vi "DAQinfo.vi"() -> (0 "错误？":bool, 1 "错误信息":string, 2 "DaqSn":string, 3 "DeviceNO":tag)   [LabVIEW 2010]
uses:
  C:/Program Files (x86)/National Instruments/LabVIEW 2010/resource/objmgr/daqmx.rc
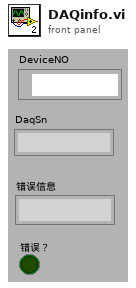
[diagram p1: front panel]
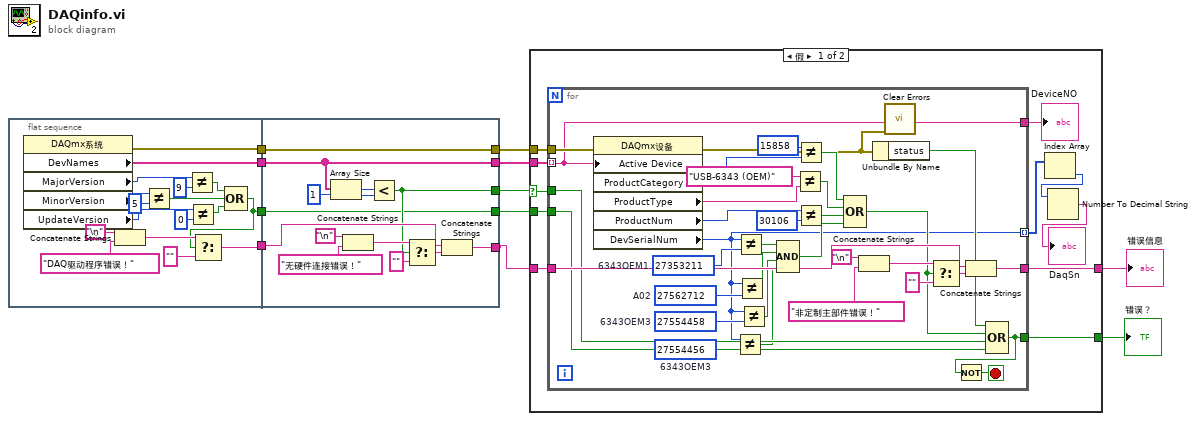
[diagram p0: block diagram]
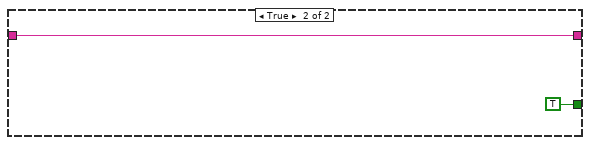
[diagram p2: hidden frame]
diagram:
  n1 = flat-sequence {
    tunnel: [w28] -> w11
    tunnel: [w21] -> w10
    tunnel: [w13] -> w8
    tunnel: [w12] -> w5
    tunnel: [w38] -> w3
    tunnel: [w41] -> w9
    tunnel: w11 -> [w41]
    tunnel: w10 -> [w38]
    tunnel: w8 -> [w33]
    tunnel: [w32] -> w7
    tunnel: [w30] -> w2
    tunnel: [w29] -> w4
    tunnel: w5 -> [w29]
    frame #0 {
      n2 = property class="DAQmx系统"() -> (error out=w28:errorcluster, "DevNames"=w21:tag[], "MajorVersion"=w27:u32, "MinorVersion"=w24:u32, "UpdateVersion"=w22:u32)  [unwired: 2 in, 1 out]
      n3 = Concatenate Strings("\n", "DAQ驱动程序错误！" ("消息")) -> (w15:string)
      n4 = Not Equal?(x=w24, y=u32 5) -> (x != y?=w19:bool)
      n5 = Not Equal?(x=w27, y=u32 9) -> (x != y?=w20:bool)
      n6 = Not Equal?(x=w22, y=u32 0) -> (x != y?=w18:bool)
      n7 = Compound Arithmetic op=OR(w20, w19, w18) -> (w12:bool)
      n8 = Select(t=w15, s=w12, f="") -> (s? t:f=w13:string)
    }
    frame #1 {
      n9 = Array Size(array=w38) -> (size(s)=w39:i32)
      n10 = Concatenate Strings("\n", "无硬件连接错误！" ("消息")) -> (w36:string)
      n11 = Less?(x=w39, y=1) -> (x < y?=w30:bool)
      n12 = Select(t=w36, s=w30, f="") -> (s? t:f=w34:string)
      n13 = Concatenate Strings(w33, w34) -> (w32:string)
    }
  }
  n14 = case shown="假" w2 {
    selector: w2 -> [w45 _]
    tunnel: w9 -> [w52 _]
    tunnel: w7 -> [w50 w89]
    tunnel: [w49 w89] -> w6
    tunnel: w4 -> [w48 _]
    tunnel: [w47 TRUE] -> w1
    tunnel: w3 -> [w46 _]
    frame False {
      n15 = for {
        tunnel: w52 -> [w87]
        tunnel: [w58] -> w51
        tunnel: w50 -> [w71]
        tunnel: [w70] -> w49
        tunnel: w45 -> [w69]
        tunnel: w48 -> [w68]
        tunnel: [w56] -> w47
        tunnel: w46 -> [w58] mode=indexing
        tunnel: [w53] -> w44 mode=indexing
        stop <- w57 stop-if-true
        w55 = u32 27554456  # 6343OEM3
        w59 = u32 27554458  # 6343OEM3
        w64 = u32 27562712  # A02
        w77 = u32 27353211  # 6343OEM1
        n16 = property class="DAQmx设备"(error in=w87, "Active Device"=w58) -> (error out=w65:errorcluster, "ProductCategory"=w86:i32, "ProductType"=w83:string, "ProductNum"=w81:u32, "DevSerialNum"=w53:u32)  [unwired: 1 in, 1 out]
        n17 = Not Equal?(x=w53, y=w55) -> (x != y?=w54:bool)
        n18 = Not Equal?(x=w53, y=w77) -> (x != y?=w62:bool)
        n19 = Not Equal?(x=w53, y=w64) -> (x != y?=w61:bool)
        n20 = Not Equal?(x=w53, y=w59) -> (x != y?=w60:bool)
        n21 = Compound Arithmetic op=AND(w62, w61, w60, w54) -> (w63:bool)
        n22 = Not Equal?(x="USB-6343 (OEM)" ("字符串"), y=w83) -> (x != y?=w79:bool)
        n23 = Not Equal?(x=15858, y=w86) -> (x != y?=w80:bool)
        n24 = Not Equal?(x=w81, y=u32 30106 ("DevSerialNum")) -> (x != y?=w78:bool)
        n25 = Compound Arithmetic op=OR(w80, w79, w78, w63) -> (w67:bool)
        n26 = Concatenate Strings("\n", "非定制主部件错误！" ("消息")) -> (w75:string)
        n27 = Unbundle By Name(w65) -> ("status"=w66:bool)
        n28 = call <vilib>:"Clear Errors.vi"("error in (no error)"=w65) -> ()  [unwired: 6 in, 1 out]
        n29 = Select(t=w75, s=w67, f="") -> (s? t:f=w73:string)
        n30 = Concatenate Strings(w71, w73) -> (w70:string)
        n31 = Compound Arithmetic op=OR(w66, w67, w69, w68) -> (w56:bool)
        n32 = Not(x=w56) -> (.not. x?=w57:bool)
      }
      "DeviceNO" <- w51
      n33 = Index Array(array=w44) -> (element=w43:u32)  [unwired: 1 in]
      n34 = Number To Decimal String(number=w43) -> (decimal integer string=→"DaqSn":string)  [unwired: 1 in]
    }
    frame True {
    }
  }
  "错误信息" <- w6
  "错误？" <- w1
